vi "test Non Match Fails The Test - Use slash codes in result.vi"(8 "error in (no error)":errorcluster, 11 "TestCase in":refnum<class "String Regex Test Case.lvclass">) -> (0 "error out":errorcluster, 3 "TestCase out":refnum<class "String Regex Test Case.lvclass">)   [LabVIEW 2015, in "String Regex Test Case.lvclass"]
uses:
  String Regex Test Case.lvclass
  <vilib>/addons/_JKI Toolkits/VI Tester/TestCase.llb/TestCase.lvclass
  VITAC.lvlib
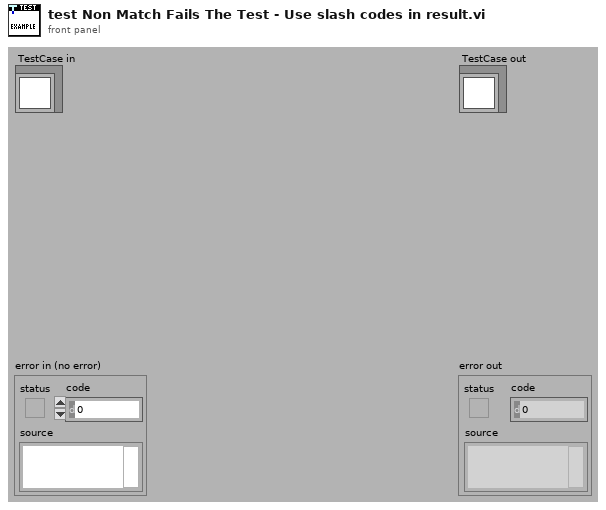
[diagram p1: front panel]
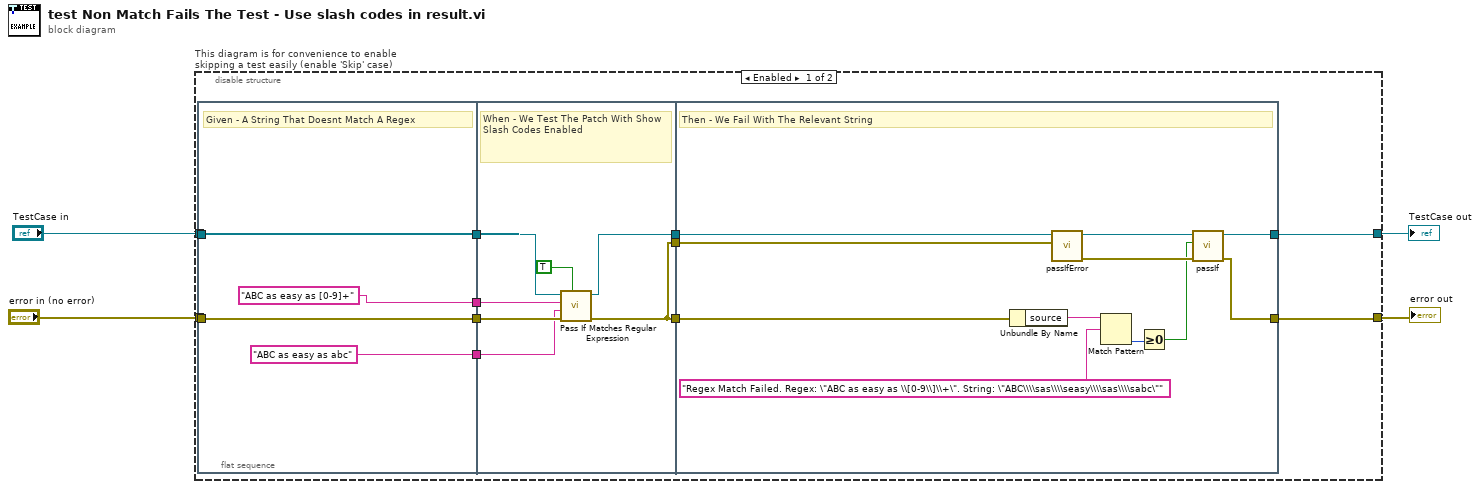
[diagram p0: block diagram]
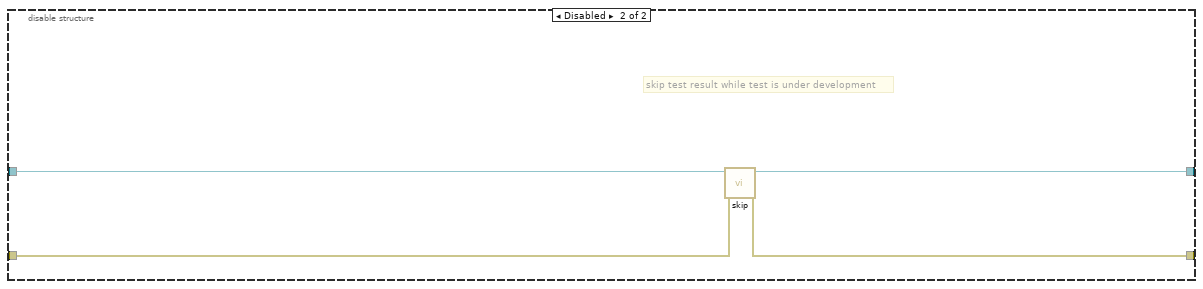
[diagram p2: hidden frame]
diagram:
  n1 = disable-structure "This diagram is for convenience to enable skipping a test easily (enable 'Skip' case)" shown="Enabled" {
    disable-tunnel: "TestCase in" -> [w12 w41]
    disable-tunnel: [w10 w39] -> w1
    disable-tunnel: [w9 w40] -> w3
    disable-tunnel: "error in (no error)" -> [w11 w38]
    frame Enabled {
      n2 = flat-sequence {
        tunnel: w11 -> [w18]
        tunnel: w12 -> [w19]
        tunnel: [w19] -> w15
        tunnel: [w18] -> w14
        tunnel: ["ABC as easy as abc" ("actual")] -> w8
        tunnel: ["ABC as easy as [0-9]+" ("actual")] -> w7
        tunnel: [w24] -> w13
        tunnel: w15 -> [w25]
        tunnel: w14 -> [w26]
        tunnel: w8 -> [w23]
        tunnel: w7 -> [w22]
        tunnel: [w21] -> w6
        tunnel: [w21] -> w5
        tunnel: w13 -> [w37]
        tunnel: [w31] -> w10
        tunnel: [w28] -> w9
        tunnel: w6 -> [w35]
        tunnel: w5 -> [w34]
        frame #0 {
          # "Given - A String That Doesnt Match A Regex"
        }
        frame #1 {
          # "When - We Test The Patch With Show Slash Codes Enabled"
          n3 = call "Pass If Matches Regular Expression.vi"("Show \\ codes (F)"=TRUE ("Show \\ codes (F)"), "error in (no error)"=w26, "actual"=w23, "regular expression"=w22, "TestCase in"=w25) -> ("error out"=w21:errorcluster, "TestCase out"=w24:refnum<class "String Regex Test Case.lvclass">)  [unwired: 5 in]
        }
        frame #2 {
          # "Then - We Fail With The Relevant String"
          n4 = Unbundle By Name(w34) -> ("source"=w33:string)
          n5 = call-dynamic "passIfError.vi"("error"=w35, "TestCase in"=w37) -> ("error out"=w30:errorcluster, "TestCase out"=w36:refnum<class "String Regex Test Case.lvclass">)  [unwired: 8 in]
          n6 = Match Pattern(string=w33, regular expression="Regex Match Failed. Regex: \"ABC as easy as \\[0-9\\]\\+\". String: \"ABC\\\\sas\\\\seasy\\\\sas\\\\sabc\"" ("actual")) -> (offset past match=w32:i32)  [unwired: 1 in, 3 out]
          n7 = Greater Or Equal To 0?(x=w32) -> (x >= 0?=w29:bool)
          n8 = call-dynamic "passIf.vi"("error in (no error)"=w30, "pass"=w29, "TestCase in"=w36) -> ("error out"=w28:errorcluster, "TestCase out"=w31:refnum<class "String Regex Test Case.lvclass">)  [unwired: 7 in]
        }
      }
    }
    frame Disabled {
      # "skip test result while test is under development"
      n9 = call <vilib>:"skip.vi"("error in (no error)"=w38, "TestCase in"=w41) -> ("error out"=w40:errorcluster, "TestCase out"=w39:refnum<class "String Regex Test Case.lvclass">)  [unwired: 8 in]
    }
  }
  "error out" <- w3
  "TestCase out" <- w1
